vi "Handle Active State.vi"(0 "reference in":refnum<class "PM_Group.lvclass">, 11 "error in (no error)":errorcluster) -> (4 "reference out":refnum<class "PM_Group.lvclass">, 15 "error out":errorcluster)   [LabVIEW 2019, in "PM_Group.lvclass"]
uses:
  PM_Group.lvclass
  C:/Users/H4001/Documents/GitHub/H4000/src/Device_class/Device.lvclass
  PM_Group.lvclass/PM_Group.ctl
  AI_class/AI.lvclass/AI.ctl
  AnalogComparator_class/AnalogComparator.lvclass/AnalogComparator.ctl
  Engine_1DO_2DI_class/Engine_1DO_2DI.lvclass/Engine_1DO_2DI.ctl
  Device_class/Device.lvclass/Device.ctl
  AI_class/Get_Values.vi
  Engine_1DO_2DI_class/TupnOn.vi
  Engine_1DO_2DI_class/GetEngineState.vi
  Device_class/GetFPGA.vi
  AnalogComparator_class/GetStatus.vi
  Engine_1DO_2DI_class/Engine_1DO_2DI.lvclass
  FPGA_API_class/Write Do.vi
  Engine_1DO_2DI_class/TupnOff.vi
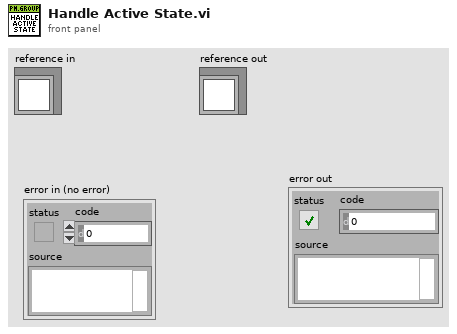
[diagram p1: front panel]
types:
  T1 = typedef "State PMG.ctl" = enum16{"NOT READY", "IDLE", "ACTIVE", "ERROR"}
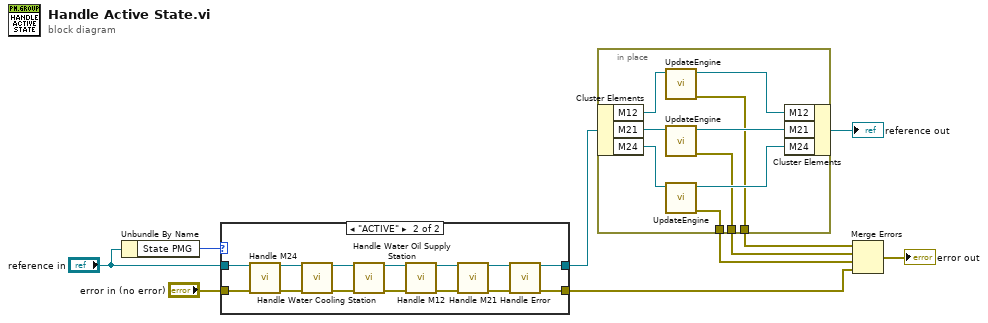
[diagram p0: block diagram]
diagram:
  n1 = Unbundle By Name("reference in") -> ("State PMG"=w10:T1)
  n2 = case shown="\"ACTIVE\"" w10 {
    tunnel: "reference in" -> [w12 w26]
    tunnel: [w12 w13] -> w7
    tunnel: "error in (no error)" -> [w11 w24]
    tunnel: [w11 w14] -> w1
    frame Default {
    }
    frame "ACTIVE" {
      n3 = call "Handle M24.vi"("reference in"=w26, "error in (no error)"=w24) -> ("reference out"=w20:refnum<class "PM_Group.lvclass">, "error out"=w19:errorcluster)  [unwired: 12 in]
      n4 = call "Handle Water Cooling Station.vi"("reference in"=w20, "error in (no error)"=w19) -> ("reference out"=w21:refnum<class "PM_Group.lvclass">, "error out"=w22:errorcluster)  [unwired: 12 in]
      n5 = call "Handle Water Oil Supply Station.vi"("reference in"=w21, "error in (no error)"=w22) -> ("reference out"=w25:refnum<class "PM_Group.lvclass">, "error out"=w23:errorcluster)  [unwired: 12 in]
      n6 = call "Handle M12.vi"("reference in"=w25, "error in (no error)"=w23) -> ("reference out"=w17:refnum<class "PM_Group.lvclass">, "error out"=w18:errorcluster)  [unwired: 12 in]
      n7 = call "Handle M21.vi"("reference in"=w17, "error in (no error)"=w18) -> ("reference out"=w16:refnum<class "PM_Group.lvclass">, "error out"=w15:errorcluster)  [unwired: 12 in]
      n8 = call "Handle Error.vi"("reference in"=w16, "error in (no error)"=w15) -> ("reference out"=w13:refnum<class "PM_Group.lvclass">, "error out"=w14:errorcluster)  [unwired: 12 in]
    }
  }
  n9 = in-place {
    in-place-border: [w29] -> w5
    in-place-border: [w28] -> w4
    in-place-border: [w27] -> w3
    n10 = in-place-cluster #1(w7) -> ("M12"=w35:refnum<class "Engine_1DO_2DI.lvclass">, "M21"=w33:refnum<class "Engine_1DO_2DI.lvclass">, "M24"=w32:refnum<class "Engine_1DO_2DI.lvclass">)
    n11 = call "UpdateEngine.vi"("Pump_1AI_1DO_2DI in"=w35) -> ("error out"=w29:errorcluster, "Pump_1AI_1DO_2DI out"=w34:refnum<class "Engine_1DO_2DI.lvclass">)  [unwired: 9 in]
    n12 = call "UpdateEngine.vi"("Pump_1AI_1DO_2DI in"=w33) -> ("error out"=w28:errorcluster, "Pump_1AI_1DO_2DI out"=w31:refnum<class "Engine_1DO_2DI.lvclass">)  [unwired: 9 in]
    n13 = call "UpdateEngine.vi"("Pump_1AI_1DO_2DI in"=w32) -> ("error out"=w27:errorcluster, "Pump_1AI_1DO_2DI out"=w30:refnum<class "Engine_1DO_2DI.lvclass">)  [unwired: 9 in]
    n14 = in-place-cluster #1("M12"=w34, "M21"=w31, "M24"=w30) -> (→"reference out":refnum<class "PM_Group.lvclass">)
  }
  n15 = Merge Errors(w5, w4, w3, w1) -> (→"error out":errorcluster)
